vi "Result Status.vi"(8 "error in (no error)":errorcluster, 11 "PQ Result in":refnum<class "PQ Result.lvclass">) -> (0 "error out":errorcluster, 2 "Result Status":T1, 3 "PQ Result out":refnum<class "PQ Result.lvclass">)   [LabVIEW 2015, in "PQ Result.lvclass"]
uses:
  PQ Result.lvclass
  Result Status.ctl
  PQ Result.lvclass/PQ Result.ctl
  Connection/libpq.dll
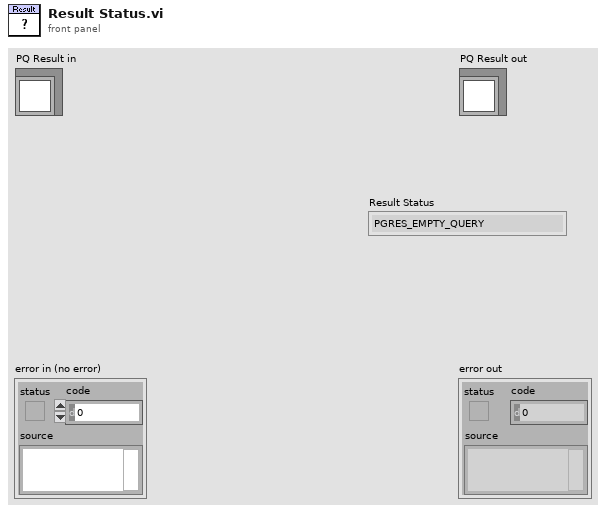
[diagram p1: front panel]
types:
  T1 = typedef "PQ Result.lvclass/Result Status.ctl" = enum32{"PGRES_EMPTY_QUERY", "PGRES_COMMAND_OK", "PGRES_TUPLES_OK", "PGRES_COPY_OUT", "PGRES_COPY_IN", "PGRES_BAD_RESPONSE", "PGRES_NONFATAL_ERROR", "PGRES_FATAL_ERROR", "PGRES_COPY_BOTH", "PGRES_SINGLE_TUPLE"}
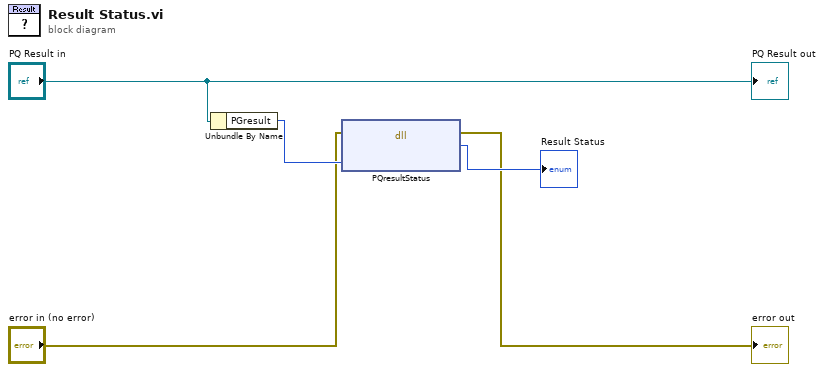
[diagram p0: block diagram]
diagram:
  n1 = Unbundle By Name("PQ Result in") -> ("PGresult"=w4:u32)
  n2 = dll-call lib="C:/PQ/Connection/libpq.dll" fn="PQresultStatus" ("libpq.*:PQstatus")(error in="error in (no error)", "PGresult"=w4) -> (error out=→"error out":errorcluster, "PQstatus"=→"Result Status":u32)  [unwired: 3 in, 1 out]
  "PQ Result out" <- "PQ Result in"
